vi "From Pythonic - Integer.vi"(4 "Pythonic Value":string) -> (1 "Integer":i64)   [LabVIEW 2012, in "OPI.lvclass"]
doc: "Convert pythonic values into LabVIEW data. This method can be helpfull to convert elements of tuples or dictionaries.\n\nReturn an integer - LabVIEW I64 representation."
uses:
  OPI.lvclass
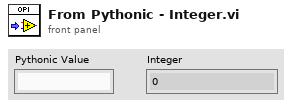
[diagram p1: front panel]
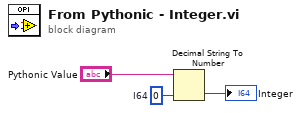
[diagram p0: block diagram]
diagram:
  w1 = i64 0  # I64
  n1 = Decimal String To Number(string="Pythonic Value", default (0L)=w1) -> (number=→"Integer":i64)  [unwired: 1 in, 1 out]
